vi "Flash_replace.vi"(7 "DUT":string, 8 "error in":errorcluster, 10 "Array":string[](array[string])=["COM50", "D:\\Users\\A. Halstesd Evander\\Documents\\DTU_Manual_Flash\\Info\\Configuration\\RX01_DTU_N58_Application_0_0_10.pac", "E:\\Users\\A. Halstesd Evander\\Downloads\\RESEARCHDOWNLOAD_R22.19.1701\\RESEARCHDOWNLOAD_R22.19.1701\\Bin\\CmdDloader.exe", "F:\\Users\\A. Halstesd Evander\\Downloads\\RESEARCHDOWNLOAD_R22.19.1701\\RESEARCHDOWNLOAD_R22.19.1701\\Bin\\result.txt"], 11 "file path (use dialog)":path) -> (0 "error out":errorcluster)   [LabVIEW 2024, in "Neoway_flashing.lvlib"]
uses:
  Neoway_flashing.lvlib
  Launcher/Launcher_DTU.lvlib
panel:
  out "String":string
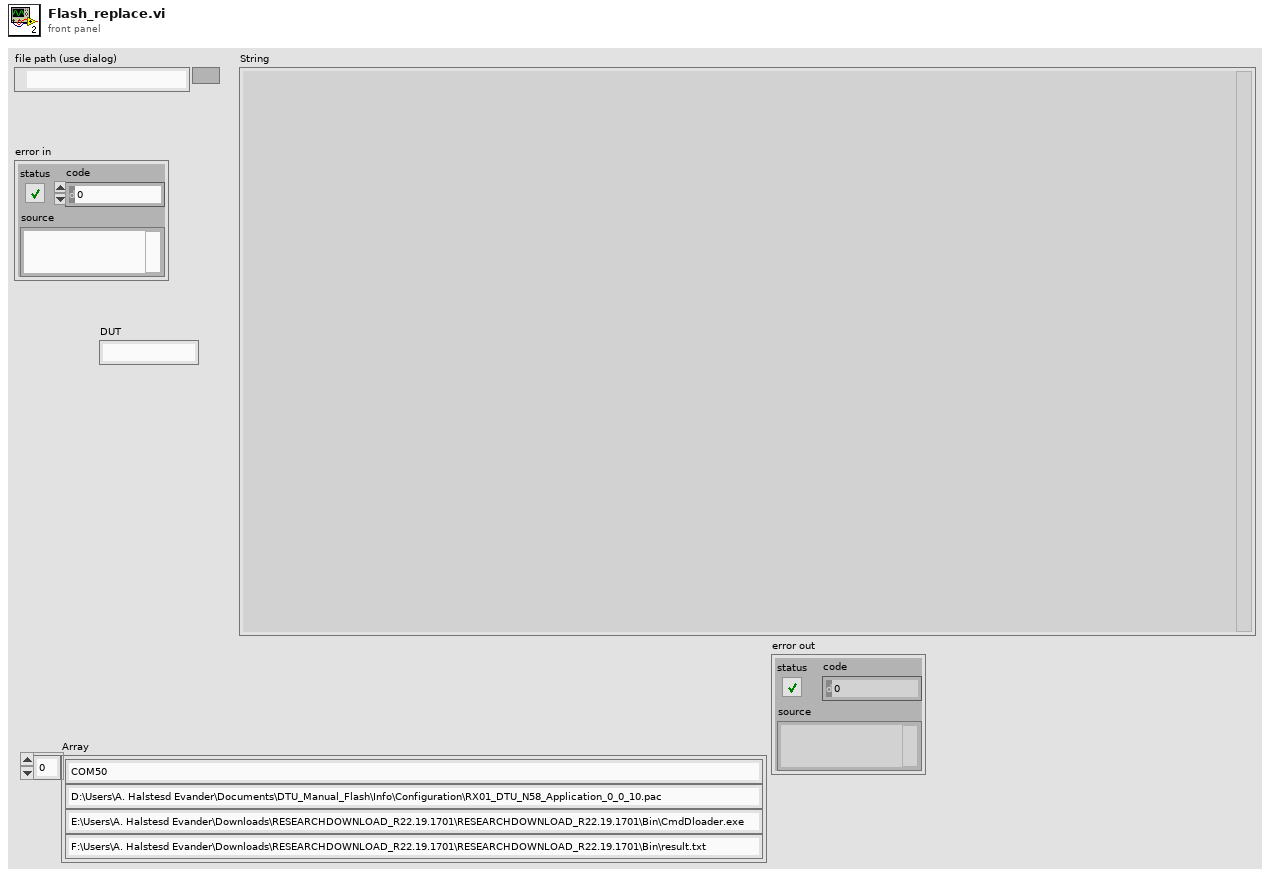
[diagram p1: front panel]
types:
  T1 = enum16{"Read", "Write", "All_sections", "All_values", "Remove key&section"}
  T2 = enum16{"open", "replace", "create", "open or create", "replace or create", "replace or create with confirmation"}
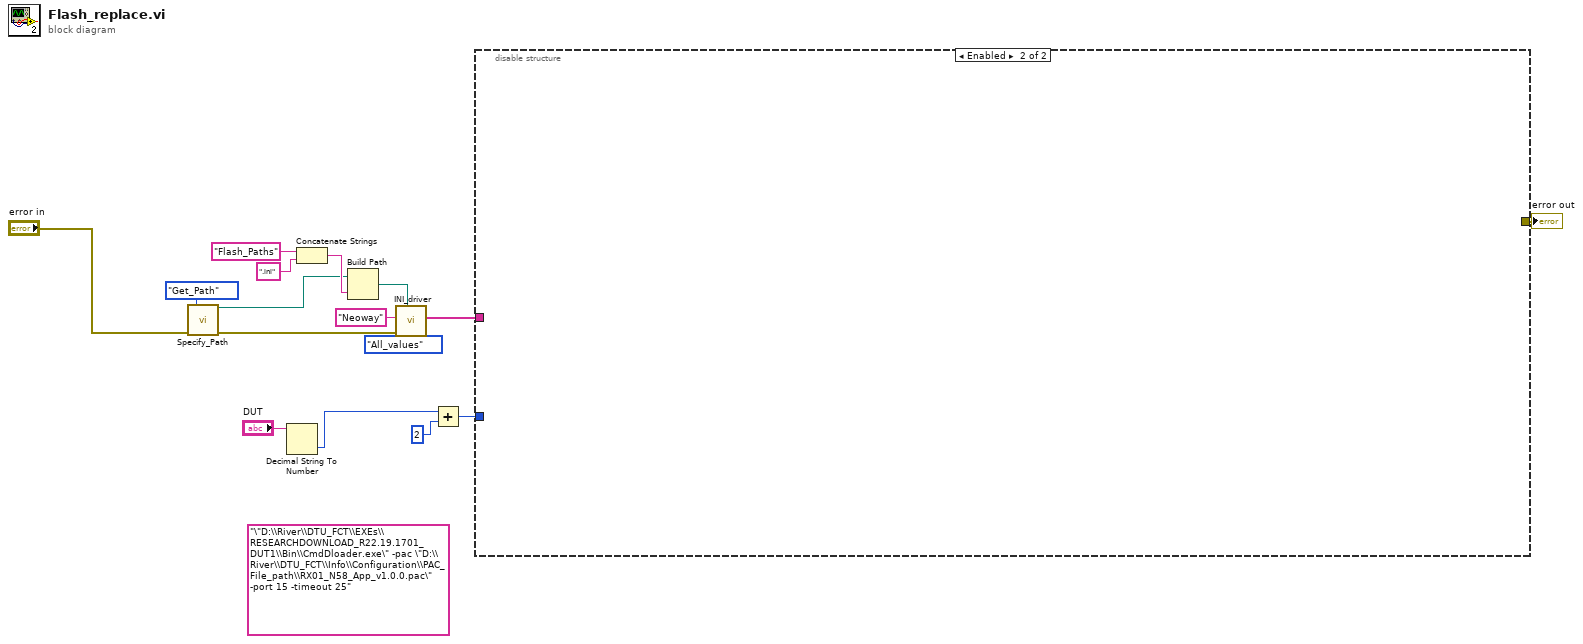
[diagram p0: block diagram]
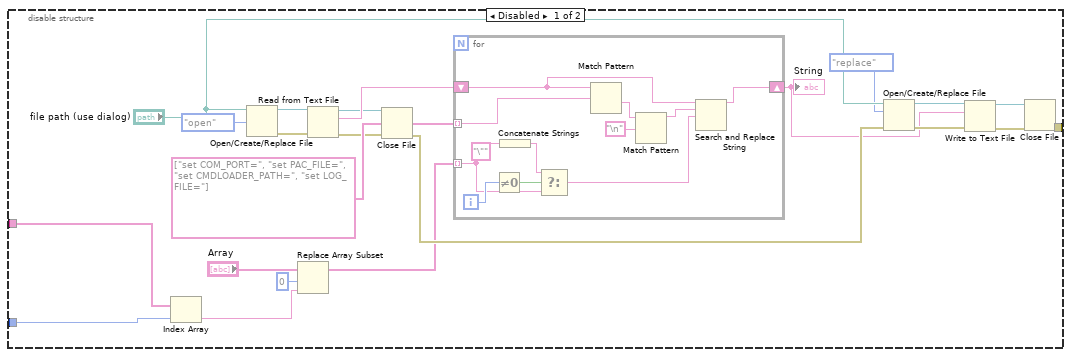
[diagram p2: hidden frame]
diagram:
  (unwired) "\"D:\\River\\DTU_FCT\\EXEs\\RESEARCHDOWNLOAD_R22.19.1701_DUT1\\Bin\\CmdDloader.exe\" -pac \"D:\\River\\DTU_FCT\\Info\\Configuration\\PAC_File_path\\RX01_N58_App_v1.0.0.pac\" -port 15 -timeout 25"
  n1 = call "Specify_Path.vi"("Path_Enum"=enum16{"Find_Path", "Get_Path"}."Get_Path", "error in (no error)"="error in") -> ("Configurations"=w7:path, "error out"=w11:errorcluster)  [unwired: 6 in, 6 out]
  n2 = Decimal String To Number(string="DUT") -> (number=w1:i32)  [unwired: 2 in, 1 out]
  n3 = Concatenate Strings("Flash_Paths" ("string"), ".ini" ("string")) -> (w13:string)
  n4 = Build Path(base path=w7, name or relative path=w13) -> (appended path=w12:path)
  n5 = call "INI_driver.vi"("Enum"=T1."All_values", "instrument file path"=w12, "error in (no error)"=w11, "Section"="Neoway") -> ("Values out"=w5:string[])  [unwired: 4 in, 3 out]
  n6 = Add(x=w1, y=2) -> (x+y=w3:i32)
  n7 = disable-structure shown="Enabled" {
    disable-tunnel: [w22 _] -> w16
    disable-tunnel: w5 -> [w21 _]
    disable-tunnel: w3 -> [w17 _]
    frame Disabled {
      n8 = Index Array(array=w21, index=w17) -> (element=w18:string)
      n9 = Open/Create/Replace File(file path (use dialog)="file path (use dialog)", operation (0:open)=T2."open") -> (refnum out=w36:refnum<file>, error out=w37:errorcluster)  [unwired: 4 in, 1 out]
      n10 = Replace Array Subset(array="Array", new element=w18, index=0) -> (w20:string[])
      n11 = Read from Text File(file (use dialog)=w36, error in=w37) -> (refnum out=w31:refnum<file>, text=w34:string, error out=w32:errorcluster)  [unwired: 2 in, 1 out]
      n12 = Close File(refnum=w31, error in=w32) -> (error out=w28:errorcluster)  [unwired: 1 out]
      n13 = for {
        tunnel: string[] ["set COM_PORT=", "set PAC_FILE=", "set CMDLOADER_PATH=", "set LOG_FILE="] -> [w49] mode=indexing
        shift-right: [w42] -> w23
        shift-left: w34 -> [w48]
        tunnel: w20 -> [w44] mode=indexing
        i -> [w46]
        (unwired) "\"" ("string")
        n14 = Not Equal To 0?(x=w46) -> (x != 0?=w47:bool)
        n15 = Concatenate Strings(w44) -> (w45:string)
        n16 = Select(t=w45, s=w47, f=w44) -> (s? t:f=w43:string)
        n17 = Match Pattern(string=w48, regular expression=w49) -> (after substring=w41:string)  [unwired: 1 in, 3 out]
        n18 = Match Pattern(string=w41, regular expression="\n") -> (before substring=w39:string)  [unwired: 1 in, 3 out]
        n19 = Search and Replace String(input string=w48, search string=w39, replace string=w43) -> (result string=w42:string)  [unwired: 5 in, 3 out]
      }
      "String" <- w23
      n20 = Open/Create/Replace File(file path (use dialog)="file path (use dialog)", error in=w28, operation (0:open)=T2."replace") -> (refnum out=w27:refnum<file>, error out=w26:errorcluster)  [unwired: 3 in, 1 out]
      n21 = Write to Text File(file (use dialog)=w27, text=w23, error in=w26) -> (refnum out=w24:refnum<file>, error out=w25:errorcluster)  [unwired: 1 in, 1 out]
      n22 = Close File(refnum=w24, error in=w25) -> (error out=w22:errorcluster)  [unwired: 1 out]
    }
    frame Enabled {
    }
  }
  "error out" <- w16
